vi "Save Bundle Definitions.vi"(8 "error in (no error)":errorcluster, 11 "Bundle Builder in":refnum<class "Bundle Builder.lvclass">) -> (0 "error out":errorcluster, 3 "Bundle Builder out":refnum<class "Bundle Builder.lvclass">)   [LabVIEW 2020, in "Bundle Builder.lvclass"]
uses:
  Bundle Builder.lvclass
  Bundle Builder.lvclass/Bundle Builder.ctl
  C:/Users/chihong/Documents/Repos/StsCustomBundleBuilder/StsCustomBundleBuilder/StsCustomBundleBuilderLib/StsCustomBundleBuilderLib.dll
  StsCustomBundleBuilderLib/StsCustomBundleBuilderLib.dll
  <vilib>/Utility/error.llb/Error Cluster From Error Code.vi
  <vilib>/ErrorRing/Error Ring.xnode
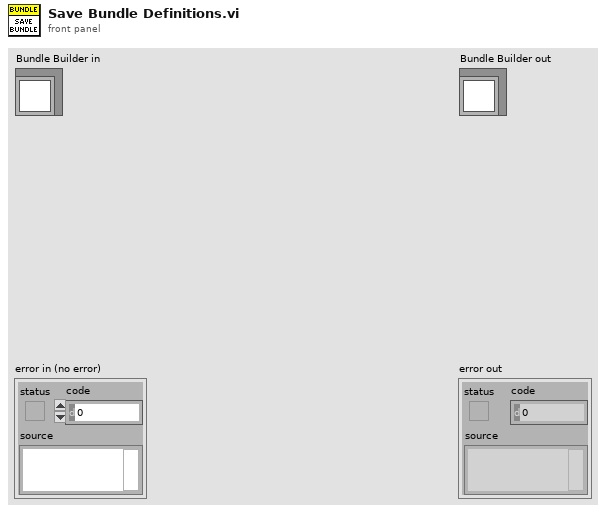
[diagram p1: front panel]
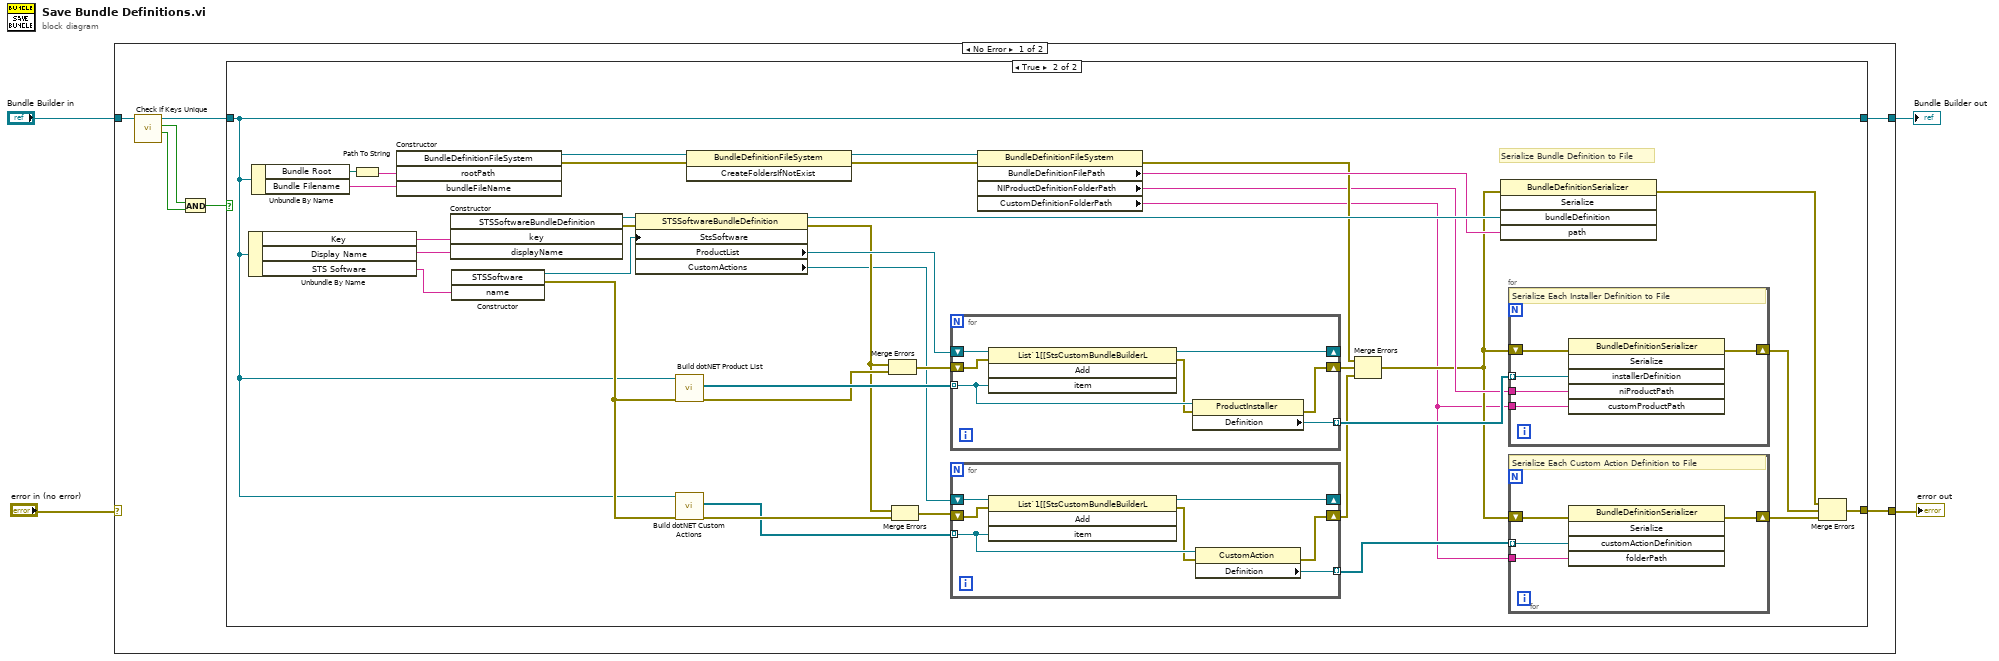
[diagram p0: block diagram]
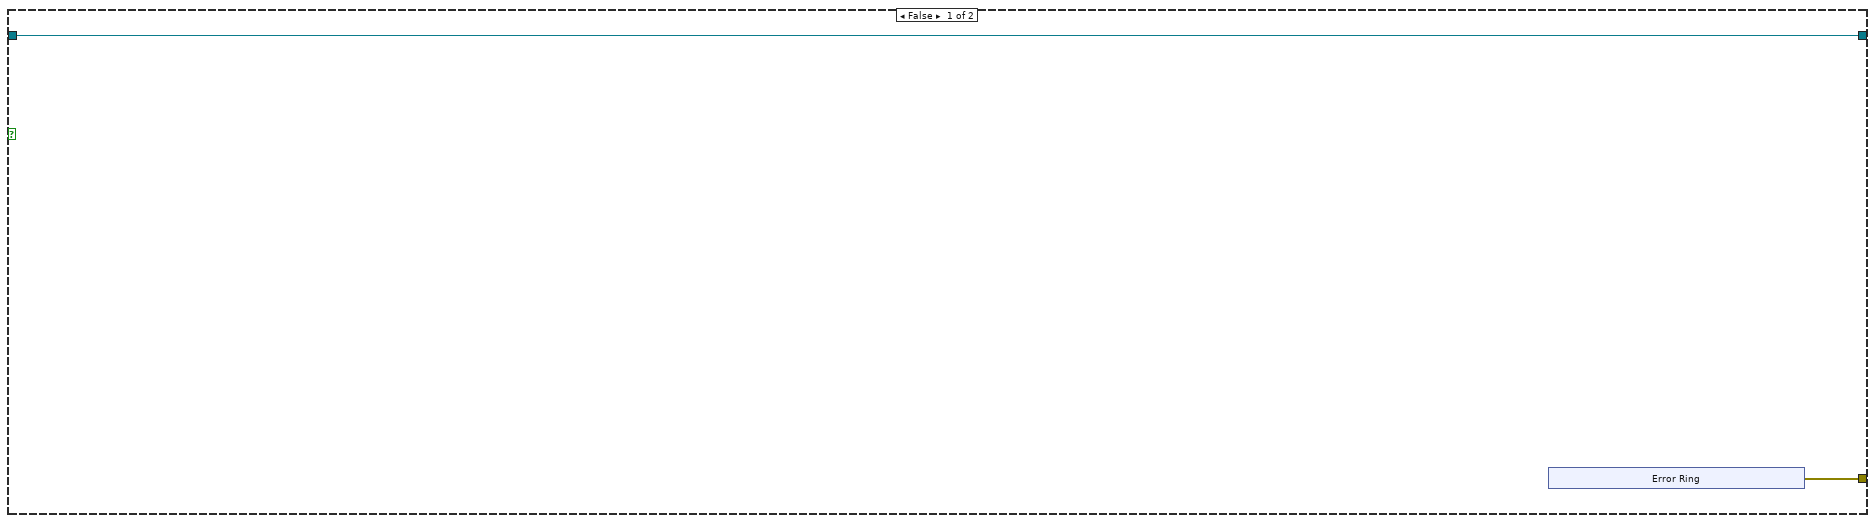
[diagram p2: hidden frame]
diagram:
  n1 = case shown="No Error" "error in (no error)" {
    selector: "error in (no error)" -> [_ w81]
    tunnel: [w5 w81] -> w3
    tunnel: [w6 w80] -> w1
    tunnel: "Bundle Builder in" -> [w11 w80]
    frame No Error {
      n2 = call "Check If Keys Unique.vi"("Bundle Builder in"=w11) -> ("Custom Action Key Unique?"=w9:bool, "Product Key Unique?"=w10:bool, "Bundle Builder out"=w7:refnum<class "Bundle Builder.lvclass">)  [unwired: 7 in, 1 out]
      n3 = And(x=w10, y=w9) -> (x .and. y?=w8:bool)
      n4 = case shown="True" w8 {
        tunnel: w7 -> [w13 w22]
        tunnel: [w13 w22] -> w6
        tunnel: [w12 w23] -> w5
        frame False {
          n5 = xnode "Error Ring"() -> ("error out"=w12:errorcluster)
        }
        frame True {
          # "Serialize Bundle Definition to File"
          n6 = Unbundle By Name(w22) -> ("Key"=w52:string, "Display Name"=w51:string, "STS Software"=w50:string)
          n7 = Unbundle By Name(w22) -> ("Bundle Root"=w56:path, "Bundle Filename"=w54:string)
          n8 = Path To String(path=w56) -> (string=w55:string)
          n9 = constructor class="BundleDefinitionFileSystem"("rootPath"=w55, "bundleFileName"=w54) -> (reference out=w20:refnum<k24>, error out=w35:errorcluster)  [unwired: 3 in, 3 out]
          n10 = constructor class="STSSoftwareBundleDefinition"("key"=w52, "displayName"=w51) -> (reference out=w53:refnum<k24>, error out=w46:errorcluster)  [unwired: 3 in, 3 out]
          n11 = constructor class="STSSoftware"("name"=w50) -> (reference out=w49:refnum<k24>, error out=w44:errorcluster)  [unwired: 3 in, 2 out]
          n12 = property class="STSSoftwareBundleDefinition"(reference=w53, error in=w46, "StsSoftware"=w49) -> (reference out=w39:refnum<k24>, error out=w41:errorcluster, "ProductList"=w48:refnum<k24>, "CustomActions"=w32:refnum<k24>)
          n13 = call "Build dotNET Product List.vi"("error in (no error)"=w44, "Bundle Builder in"=w22) -> ("error out"=w45:errorcluster, "Product List"=w47:refnum<k24>[])  [unwired: 7 in, 1 out]
          n14 = call "Build dotNET Custom Actions.vi"("error in (no error)"=w44, "Bundle Builder in"=w22) -> ("error out"=w43:errorcluster, "Custom Actions"=w31:refnum<k24>[])  [unwired: 7 in, 1 out]
          n15 = invoke class="BundleDefinitionFileSystem" method="CreateFoldersIfNotExist"(reference=w20, error in=w35) -> (reference out=w19:refnum<k24>, error out=w21:errorcluster)  [unwired: 1 in, 1 out]
          n16 = Merge Errors(w41, w45) -> (w42:errorcluster)
          n17 = Merge Errors(w41, w43) -> (w33:errorcluster)
          n18 = for {
            tunnel: w47 -> [w76] mode=indexing
            shift-right: [w73] -> w40
            shift-left: w42 -> [w78]
            shift-right: [w77] -> _
            shift-left: w48 -> [w79]
            tunnel: [w75] -> w36 mode=indexing
            n19 = invoke class="List`1[[StsCustomBundleBuilderL" method="Add"(reference=w79, error in=w78, "item"=w76) -> (reference out=w77:refnum<k24>, error out=w74:errorcluster)  [unwired: 1 in, 2 out]
            n20 = property class="ProductInstaller"(reference=w76, error in=w74) -> (error out=w73:errorcluster, "Definition"=w75:refnum<k24>)  [unwired: 1 out]
          }
          n21 = for {
            tunnel: w31 -> [w64] mode=indexing
            shift-right: [w61] -> w30
            shift-left: w33 -> [w66]
            shift-right: [w65] -> _
            shift-left: w32 -> [w67]
            tunnel: [w63] -> w28 mode=indexing
            n22 = invoke class="List`1[[StsCustomBundleBuilderL" method="Add"(reference=w67, error in=w66, "item"=w64) -> (reference out=w65:refnum<k24>, error out=w62:errorcluster)  [unwired: 1 in, 2 out]
            n23 = property class="CustomAction"(reference=w64, error in=w62) -> (error out=w61:errorcluster, "Definition"=w63:refnum<k24>)  [unwired: 1 out]
          }
          n24 = property class="BundleDefinitionFileSystem"(reference=w19, error in=w21) -> (error out=w37:errorcluster, "BundleDefinitionFilePath"=w38:string, "NIProductDefinitionFolderPath"=w34:string, "CustomDefinitionFolderPath"=w27:string)  [unwired: 1 out]
          n25 = Merge Errors(w37, w40, w30) -> (w29:errorcluster)
          n26 = invoke class="BundleDefinitionSerializer" method="Serialize"(error in=w29, "bundleDefinition"=w39, "path"=w38) -> (error out=w26:errorcluster)  [unwired: 2 in, 4 out]
          n27 = for {
            tunnel: w36 -> [w72] mode=indexing
            tunnel: w34 -> [w70]
            tunnel: w27 -> [w69]
            shift-right: [w68] -> w25
            shift-left: w29 -> [w71]
            # "Serialize Each Installer Definition to File"
            n28 = invoke class="BundleDefinitionSerializer" method="Serialize"(error in=w71, "installerDefinition"=w72, "niProductPath"=w70, "customProductPath"=w69) -> (error out=w68:errorcluster)  [unwired: 2 in, 5 out]
          }
          n29 = for {
            tunnel: w28 -> [w60] mode=indexing
            tunnel: w27 -> [w58]
            shift-right: [w57] -> w24
            shift-left: w29 -> [w59]
            # "Serialize Each Custom Action Definition to File"
            n30 = invoke class="BundleDefinitionSerializer" method="Serialize"(error in=w59, "customActionDefinition"=w60, "folderPath"=w58) -> (error out=w57:errorcluster)  [unwired: 2 in, 4 out]
          }
          n31 = Merge Errors(w26, w25, w24) -> (w23:errorcluster)
        }
      }
    }
    frame Error {
    }
  }
  "error out" <- w3
  "Bundle Builder out" <- w1
